vi "lvRunVi.vi"() -> (0 "error out":errorcluster)   [LabVIEW 2014, in "lvcommonbuild.lvlib"]
uses:
  lvcommonbuild.lvlib
  <vilib>/Wiresmith Technology/LabVIEW CLI/CLI Class/CLI.lvclass
  security/lvbuildsecurity.lvlib
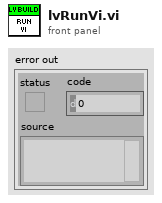
[diagram p1: front panel]
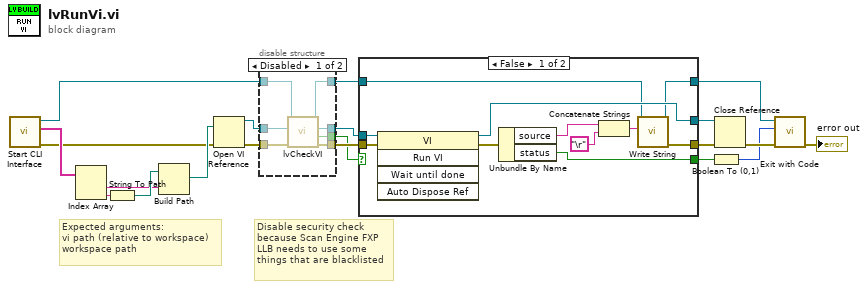
[diagram p0: block diagram]
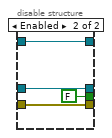
[diagram p2: hidden frame]
diagram:
  # "Disable security check\nbecause Scan Engine FXP\nLLB needs to use some\nthings that are blacklisted"
  # "Expected arguments:\nvi path (relative to workspace)\nworkspace path"
  n1 = call <vilib>:"Start CLI Interface.vi"() -> ("error out"=w13:errorcluster, "Custom Parameters"=w20:string[], "CLI out"=w6:refnum<class "CLI.lvclass">)  [unwired: 9 in]
  n2 = Index Array(array=w20) -> (element #1=w12:string, element #2=w17:string)  [unwired: 2 in]
  n3 = String To Path(string=w17) -> (path=w18:path)
  n4 = Build Path(base path=w18, name or relative path=w12) -> (appended path=w16:path)
  n5 = Open VI Reference(vi path=w16, error in (no error)=w13) -> (vi reference=w8:refnum<vi>, error out=w10:errorcluster)  [unwired: 4 in]
  n6 = disable-structure shown="Disabled" {
    disable-tunnel: w10 -> [w27 w30]
    disable-tunnel: [w26 w30] -> w9
    disable-tunnel: w8 -> [w25 w31]
    disable-tunnel: [w24 w31] -> w7
    disable-tunnel: w6 -> [w23 w28]
    disable-tunnel: [w22 FALSE ("Reject?")] -> w5
    disable-tunnel: [w21 w28] -> w4
    frame Disabled {
      n7 = call "lvCheckVI.vi"("error in (no error)"=w27, "VI Refnum"=w25, "CLI"=w23) -> ("error out"=w26:errorcluster, "Reject?"=w22:bool, "dup VI Refnum"=w24:refnum<vi>, "CLI out"=w21:refnum<class "CLI.lvclass">)  [unwired: 5 in]
    }
    frame Enabled {
    }
  }
  n8 = case shown="False" w5 {
    selector: w5 -> [_ w43]
    tunnel: w9 -> [w42 w45]
    tunnel: w7 -> [w41 w46]
    tunnel: [w36 w45] -> w15
    tunnel: [w40 w46] -> w14
    tunnel: w4 -> [w39 w44]
    tunnel: [w38 w44] -> w3
    tunnel: [w35 w43] -> w2
    frame False {
      n9 = invoke class="VI" method="Run VI"(reference=w41, error in=w42) -> (reference out=w40:refnum<vi>, error out=w37:errorcluster)  [unwired: 3 in, 3 out]
      n10 = Unbundle By Name(w37) -> ("source"=w34:string, "status"=w35:bool)
      n11 = Concatenate Strings(w34, "\r") -> (w33:string)
      n12 = call <vilib>:"Write String.vi"("Text to Write"=w33, "CLI in"=w39) -> ("error out"=w36:errorcluster, "CLI out"=w38:refnum<class "CLI.lvclass">)  [unwired: 8 in]
    }
    frame True {
    }
  }
  n13 = Boolean To (0,1)(Boolean=w2) -> (0, 1=w1:i16)
  n14 = Close Reference(reference=w14, error in (no error)=w15) -> (error out=w11:errorcluster)
  n15 = call <vilib>:"Exit with Code.vi"("error in (no error)"=w11, "Exit Code (0)"=w1, "CLI in"=w3) -> ("error out"=→"error out":errorcluster)  [unwired: 8 in]
